vi "SAOMM-Falcon2Fits.vi"(7 "ProcessedData":u8[](array[numeric])=array[17604 elements]) -> (4 "ImageBuffer":u32[][](graph), 6 "GrayLevels":u8[][](graph), 10 "MaskObjet":u8[][](graph), 12 "GeneralProperties":T3, 13 "ROIProperties":T1, 14 "ProcessedProperties":T2 {"Centroide Y" format="%.3f"; "Centroide X" format="%.3f"; "SNR" format="%.3f"; "Flux" format="%.3f"; "Seuil du masque" format="%.3f"}, 15 "MaskSeuil":u8[][](graph))   [LabVIEW 2011]
uses:
  gfitsio/cfitsio-bitpix.ctl
  gfitsio/gfitsio-write-image-subset-i32-2d.vi
  gfitsio/gfitsio.lvlib
panel:
  in  "Save?":bool
  in  "fits file":path
  out "size(s) 2":i32
  out "error out":errorcluster
  out "size(s)":i32
  out "Height":i32
  out "Width":i32
  out "ImageLen":i32
  out "BufferLen":i32
  out "ImagesIndex":i32
  in  "Path":path=path "C:/BonOMM/BonOMM-2012/SubVIs/SAOMM/ProcessedFalconImageOutput.raw"
  # "Émulation ..."
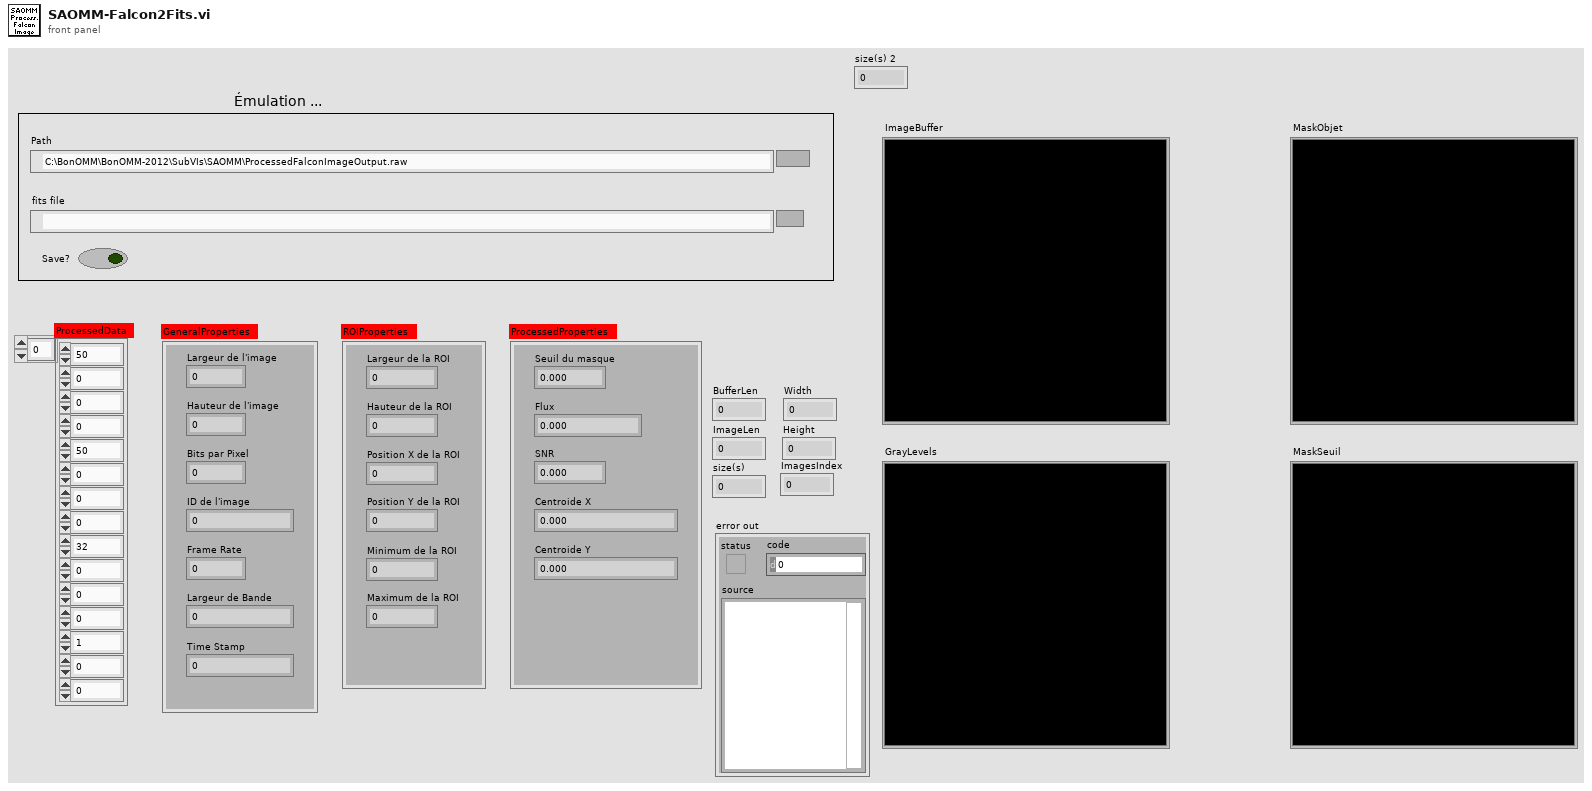
[diagram p1: front panel]
types:
  T1 = cluster{"Largeur de la ROI":u16, "Hauteur de la ROI":u16, "Position X de la ROI":u16, "Position Y de la ROI":u16, "Minimum de la ROI":u32, "Maximum de la ROI":u32}
  T2 = cluster{"Seuil du masque":dbl, "Flux":dbl, "SNR":dbl, "Centroide X":dbl, "Centroide Y":dbl}
  T3 = cluster{"Largeur de l'image":dbl, "Hauteur de l'image":dbl, "Bits par Pixel":dbl, "ID de l'image":u32, "Frame Rate":dbl, "Largeur de Bande":dbl, "Time Stamp":u64}
  T4 = enum16{"open", "open or create", "create or replace", "create", "open (read only)"}
  T5 = enum16{"open", "open or create", "create", "create or replace"}
  T6 = typedef "gfitsio.lvlib/cfitsio-bitpix.ctl" = i32
  T7 = typedef "gfitsio.lvlib/gfitsio-refnum.ctl" = refnum<k1>
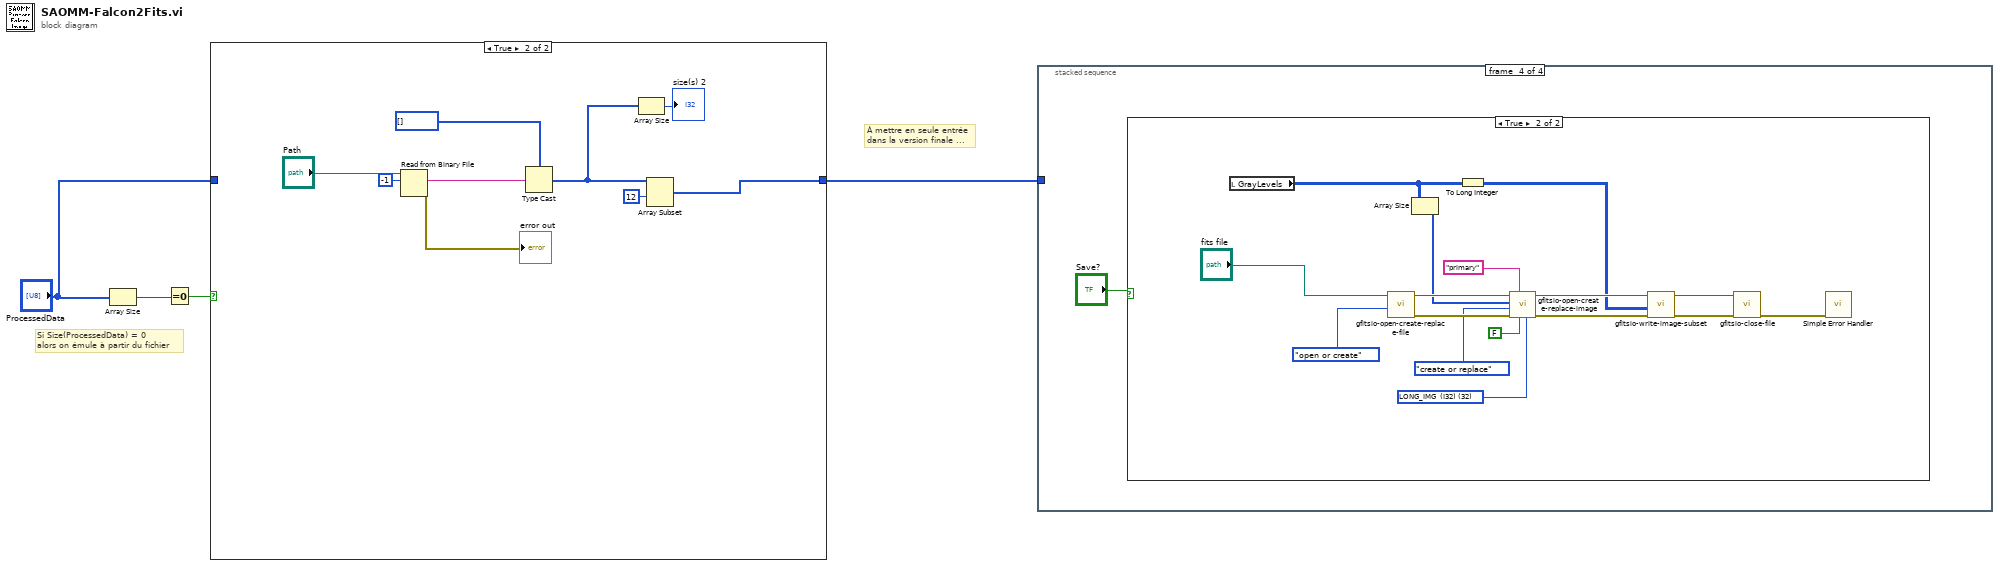
[diagram p0: block diagram]
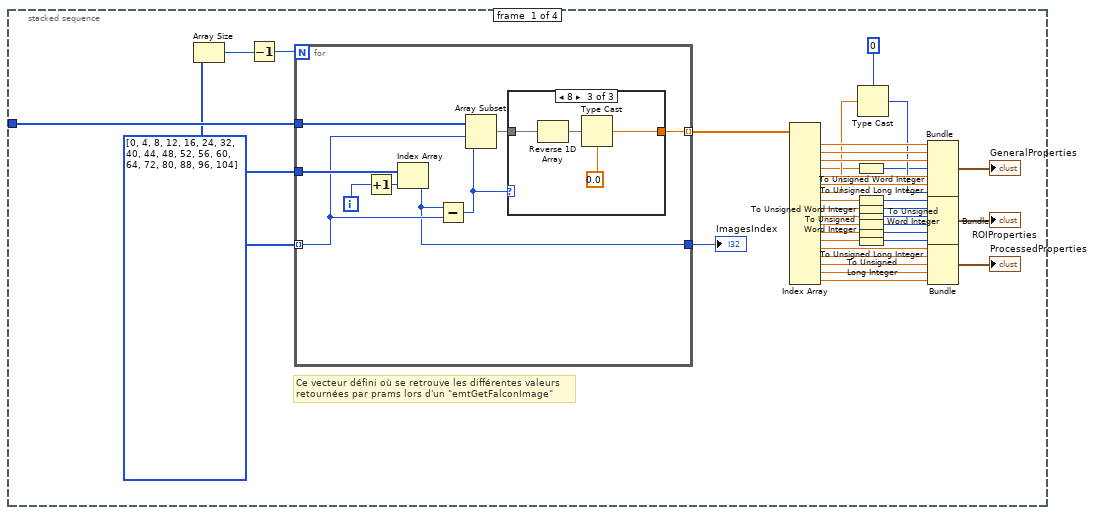
[diagram p3: hidden frame]
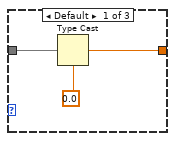
[diagram p4: hidden frame]
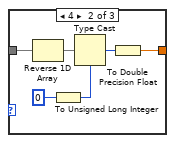
[diagram p5: hidden frame]
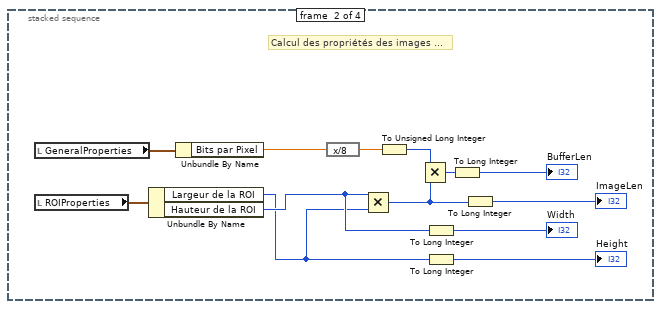
[diagram p6: hidden frame]
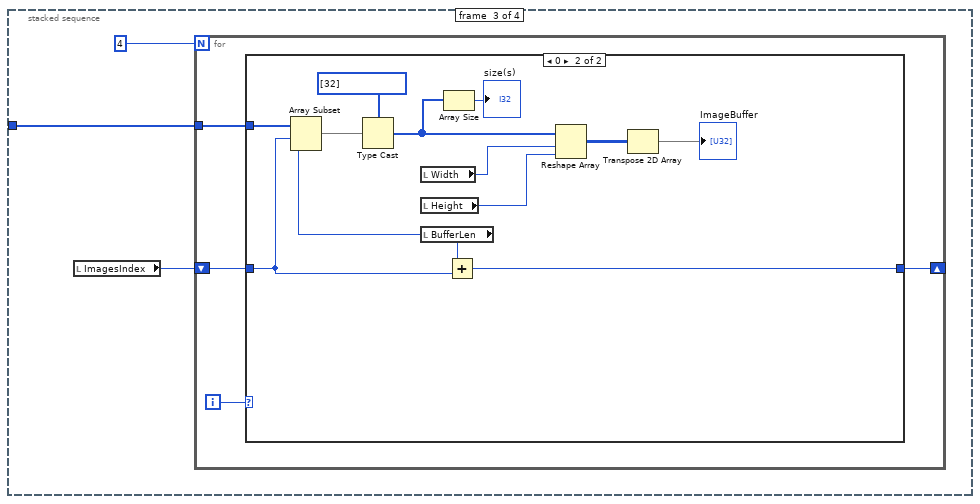
[diagram p7: hidden frame]
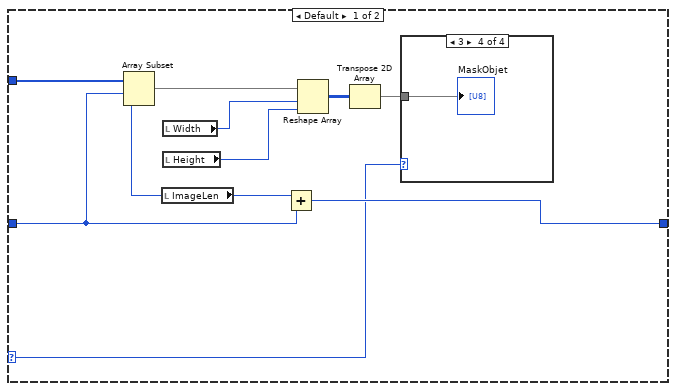
[diagram p8: hidden frame]
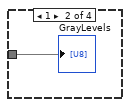
[diagram p10: hidden frame]
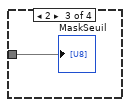
[diagram p11: hidden frame]
diagram:
  # "Si Size(ProcessedData) = 0\nalors on émule à partir du fichier"
  # "À mettre en seule entrée\ndans la version finale ..."
  n1 = Array Size(array="ProcessedData") -> (size(s)=w3:i32)
  n2 = Equal To 0?(x=w3) -> (x = 0?=w2:bool)
  n3 = case shown="True" w2 {
    tunnel: [w5 w10] -> w4
    tunnel: "ProcessedData" -> [w5 _]
    frame False {
    }
    frame True {
      n4 = Read from Binary File(10:-1 ("count (1)"), 11:"Path") -> (0:→"error out":errorcluster, 2:w12:string)  [unwired: 4 in, 2 out]
      n5 = Type Cast(type=u8[] [], x=w12) -> (*(type *) &x=w8:u8[])
      n6 = Array Size(array=w8) -> (size(s)=→"size(s) 2":i32)
      n7 = Array Subset(array=w8, index=12) -> (w10:u8[])  [unwired: 1 in]
    }
  }
  n8 = stacked-sequence {
    tunnel: w4 -> [w50 _ w88 _]
    frame #0 {
      w30 = i32[] [0, 4, 8, 12, 16, 24, 32, 40, 44, 48, 52, 56, 60, 64, 72, 80, 88, 96, 104] ("ValuesIndex")
      # "Ce vecteur défini où se retrouve les différentes valeurs\nretournées par prams lors d'un \"emtGetFalconImage\""
      n9 = Array Size(array=w30) -> (size(s)=w47:i32)
      n10 = Decrement(x=w47) -> (x-1=w48:i32)
      n11 = for {
        N: w48 -> [_]
        tunnel: w50 -> [w59]
        tunnel: w30 -> [w52] mode=indexing
        tunnel: w30 -> [w56]
        tunnel: [w53] -> w49 mode=indexing
        tunnel: [w51] -> w26
        i -> [w57]
        n12 = Increment(x=w57) -> (x+1=w58:i32)
        n13 = Index Array(array=w56, index=w58) -> (element=w51:i32)
        n14 = Subtract(x=w51, y=w52) -> (x-y=w54:i32)
        n15 = Array Subset(array=w59, index=w52, length=w54) -> (w55:u8[])
        n16 = case shown="8" w54 {
          tunnel: w55 -> [w62 w64 w69]
          tunnel: [w61 w65 w70] -> w53
          frame Default {
            n17 = Type Cast(type=0.0, x=w62) -> (*(type *) &x=w61:dbl)
          }
          frame 4 {
            n18 = Reverse 1D Array(array=w64) -> (reversed array=w63:u8[])
            n19 = To Unsigned Long Integer(number=0) -> (unsigned 32bit integer=w67:u32)
            n20 = Type Cast(type=w67, x=w63) -> (*(type *) &x=w66:u32)
            n21 = To Double Precision Float(number=w66) -> (double precision float=w65:dbl)
          }
          frame 8 {
            n22 = Reverse 1D Array(array=w69) -> (reversed array=w72:u8[])
            n23 = Type Cast(type=0.0, x=w72) -> (*(type *) &x=w70:dbl)
          }
        }
      }
      "ImagesIndex" <- w26
      n24 = Index Array(array=w49) -> (element #1=w36:dbl, element #2=w35:dbl, element #3=w34:dbl, element #4=w20:dbl, element #5=w33:dbl, element #6=w32:dbl, element #7=w29:dbl, element #8=w40:dbl, element #9=w39:dbl, element #10=w38:dbl, element #11=w37:dbl, element #12=w18:dbl, element #13=w16:dbl, element #14=w46:dbl, element #15=w45:dbl, element #16=w44:dbl, element #17=w43:dbl, element #18=w42:dbl)  [unwired: 18 in]
      n25 = To Unsigned Long Integer(number=w20) -> (unsigned 32bit integer=w21:u32)
      n26 = To Unsigned Word Integer(number=w40) -> (unsigned 16bit integer=w25:u16)
      n27 = To Unsigned Word Integer(number=w39) -> (unsigned 16bit integer=w24:u16)
      n28 = To Unsigned Word Integer(number=w38) -> (unsigned 16bit integer=w23:u16)
      n29 = To Unsigned Word Integer(number=w37) -> (unsigned 16bit integer=w22:u16)
      n30 = To Unsigned Long Integer(number=w18) -> (unsigned 32bit integer=w17:u32)
      n31 = To Unsigned Long Integer(number=w16) -> (unsigned 32bit integer=w15:u32)
      n32 = Type Cast(type=u64 0, x=w29) -> (*(type *) &x=w28:u64)
      n33 = Bundle(w36, w35, w34, w21, w33, w32, w28) -> (→"GeneralProperties":cluster{dbl, dbl, dbl, u32, dbl, dbl, u64})  [unwired: 1 in]
      n34 = Bundle(w25, w24, w23, w22, w17, w15) -> (→"ROIProperties":cluster{u16, u16, u16, u16, u32, u32})  [unwired: 1 in]
      n35 = Bundle(w46, w45, w44, w43, w42) -> (→"ProcessedProperties":cluster{dbl, dbl, dbl, dbl, dbl})  [unwired: 1 in]
    }
    frame #1 {
      # "Calcul des propriétés des images ..."
      n36 = local read "GeneralProperties"() -> (w84:T3)
      n37 = local read "ROIProperties"() -> (w85:T1)
      n38 = Unbundle By Name(w85) -> ("Largeur de la ROI"=w73:u16, "Hauteur de la ROI"=w74:u16)
      n39 = Unbundle By Name(w84) -> ("Bits par Pixel"=w83:dbl)
      n40 = expression code="x/8"(w83) -> (w78:dbl)
      n41 = Multiply(x=w74, y=w73) -> (x*y=w82:u16)
      n42 = To Unsigned Long Integer(number=w78) -> (unsigned 32bit integer=w77:u32)
      n43 = Multiply(x=w77, y=w82) -> (x*y=w76:u32)
      n44 = To Long Integer(number=w74) -> (32bit integer=→"Width":i32)
      n45 = To Long Integer(number=w73) -> (32bit integer=→"Height":i32)
      n46 = To Long Integer(number=w76) -> (32bit integer=→"BufferLen":i32)
      n47 = To Long Integer(number=w82) -> (32bit integer=→"ImageLen":i32)
    }
    frame #2 {
      n48 = local read "ImagesIndex"() -> (w87:i32)
      n49 = for {
        N: 4 -> [_]
        tunnel: w88 -> [w90]
        shift-right: [w89] -> _
        shift-left: w87 -> [w91]
        i -> [w92]
        n50 = case shown="0" w92 {
          selector: w92 -> [w95 _]
          tunnel: w91 -> [w99 w117]
          tunnel: w90 -> [w101 w111]
          tunnel: [w102 w115] -> w89
          frame Default {
            n51 = local read "ImageLen"() -> (w100:i32)
            n52 = Array Subset(array=w101, index=w99, length=w100) -> (w96:u8[])
            n53 = local read "Width"() -> (w98:i32)
            n54 = local read "Height"() -> (w97:i32)
            n55 = Add(x=w100, y=w99) -> (x+y=w102:i32)
            n56 = Reshape Array(w96, w98, w97) -> (w94:u8[][])
            n57 = Transpose 2D Array(2D array=w94) -> (transposed array=w93:u8[][])
            n58 = case shown="3" w95 {
              tunnel: w93 -> [_ w103 w104 w105]
              frame 0, Default {
                # "N'arrive jamais"
              }
              frame 1 {
                "GrayLevels" <- w103
              }
              frame 2 {
                "MaskSeuil" <- w104
              }
              frame 3 {
                "MaskObjet" <- w105
              }
            }
          }
          frame 0 {
            n59 = local read "Width"() -> (w114:i32)
            n60 = local read "Height"() -> (w113:i32)
            n61 = local read "BufferLen"() -> (w116:i32)
            n62 = Array Subset(array=w111, index=w117, length=w116) -> (w110:u8[])
            n63 = Type Cast(type=u32[] [32], x=w110) -> (*(type *) &x=w109:u32[])
            n64 = Array Size(array=w109) -> (size(s)=→"size(s)":i32)
            n65 = Add(x=w116, y=w117) -> (x+y=w115:i32)
            n66 = Reshape Array(w109, w114, w113) -> (w107:u32[][])
            n67 = Transpose 2D Array(2D array=w107) -> (transposed array=→"ImageBuffer":u32[][])
          }
        }
      }
    }
    frame #3 {
      n68 = case shown="True" "Save?" {
        frame False {
        }
        frame True {
          w128 = T6 32 items=["<invalid type>"=0, "BYTE_IMG  (U8)"=8, "SHORT_IMG  (I16)"=16, "USHORT_IMG  (U16)"=20, "LONG_IMG  (I32)"=32, "ULONG_IMG  (U32)"=40, "FLOAT_IMG  (SGL)"=-32, "DOUBLE_IMG  (DBL)"=-64] ("image data type")
          n69 = local read "GrayLevels"() -> (w125:u8[][])
          n70 = call "gfitsio-open-create-replace-file.vi"("function (open)"=T4."open or create", "file path (dialog if empty)"="fits file") -> ("error out"=w131:errorcluster, "gfits refnum"=w134:T7)  [unwired: 7 in, 1 out]
          n71 = Array Size(array=w125) -> (size(s)=w130:i32[])
          n72 = To Long Integer(number=w125) -> (32bit integer=w124:i32[][])
          n73 = call "gfitsio-open-create-replace-image.vi"("image data type"=w128, "advisory dialog? (display:T)"=FALSE, "hdu name (dialog if empty)"="primary", "error in (no error)"=w131, "function (open or create)"=T5."create or replace", "naxes"=w130, "gfits refnum"=w134) -> ("error out"=w132:errorcluster, "dup gfits refnum"=w133:T7)  [unwired: 2 in, 1 out]
          n74 = call-poly "gfitsio-write-image-subset.vi"("error in (no error)"=w132, "data"=w124, "gfits refnum"=w133) -> ("error out"=w123:errorcluster, "dup gfits refnum"=w122:T7)  [unwired: 7 in]
          n75 = call "gfitsio-close-file.vi"("error in (no error)"=w123, "gfits refnum"=w122) -> ("error out"=w121:errorcluster)  [unwired: 8 in, 1 out]
          n76 = call <vilib>:"Simple Error Handler.vi"("error in (no error)"=w121) -> ()  [unwired: 4 in, 5 out]
        }
      }
    }
  }
